vi "CVM Calcualte.vi"(9 "Load Volatage":sgl, 10 "Data":sgl[](array[numeric]), 11 "Start Index":i32) -> (3 "SummaryCVM":T1 caption="单体电压汇总" {"Voltage(E-Load)" format="%#.3f"; "DifferenceVoltage" format="%#.3f"; "Average" format="%#.3f"; "SumCVM" format="%#.3f"; "Min" format="%#.3f"; "Max" format="%#.3f"})   [LabVIEW 2020]
panel:
  # "V"
  # "V"
  # "V"
  # "V"
  # "V"
  # "V"
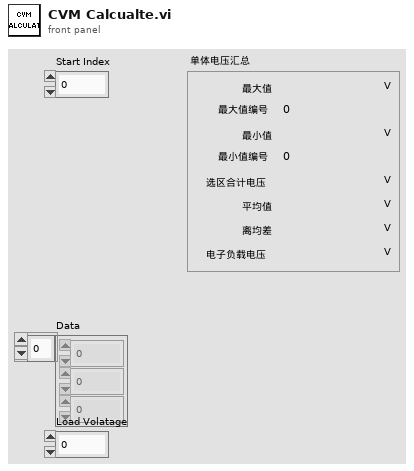
[diagram p1: front panel]
types:
  T1 = cluster{"Max":sgl, "Max_Index":i32, "Min":sgl, "Min_Index":i32, "SumCVM":sgl, "Average":sgl, "DifferenceVoltage":sgl, "Voltage(E-Load)":sgl}
  T2 = cluster{sgl, i32, sgl, i32, "数值":sgl, sgl, sgl, "Load Volatage":sgl}
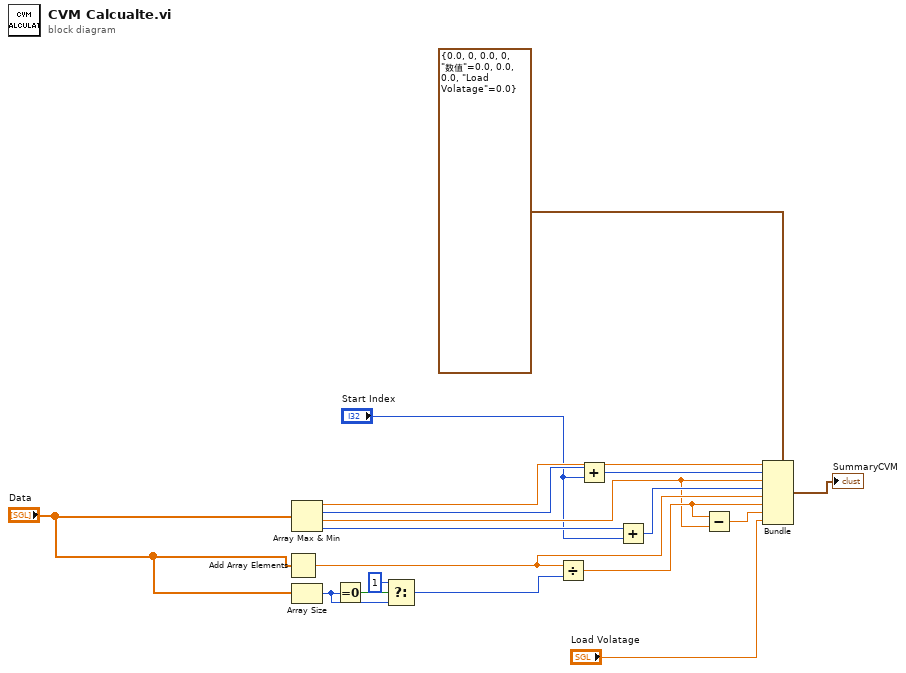
[diagram p0: block diagram]
diagram:
  n1 = Add Array Elements(numeric array="Data") -> (sum=w9:sgl)
  n2 = Array Max & Min(array="Data") -> (max value=w16:sgl, max index (indices)=w15:i32, min value=w7:sgl, min index (indices)=w14:i32)
  n3 = Array Size(array="Data") -> (size(s)=w11:i32)
  n4 = Equal To 0?(x=w11) -> (x = 0?=w13:bool)
  n5 = Select(t=1, s=w13, f=w11) -> (s? t:f=w10:i32)
  n6 = Divide(x=w9, y=w10) -> (x/y=w8:sgl)
  n7 = Add(x=w15, y="Start Index") -> (x+y=w17:i32)
  n8 = Add(x=w14, y="Start Index") -> (x+y=w18:i32)
  n9 = Subtract(x=w8, y=w7) -> (x-y=w6:sgl)
  n10 = Bundle(cluster=T2 {0.0, 0, 0.0, 0, "数值"=0.0, 0.0, 0.0, "Load Volatage"=0.0} ("簇"), w16, w17, w7, w18, "数值"=w9, w8, w6, "Load Volatage"="Load Volatage") -> (→"SummaryCVM":T2)
